vi "Push Digital.vi"(9 "Sample count":i32=8192, 10 "digital_samples":u64[](array[numeric]), 11 "ADALM2000 Handler":u32 caption="Instrument Handle Out") -> (3 "ADALM2000 Handler 2":u32 caption="Instrument Handle Out")   [LabVIEW 2015]
uses:
  libm2k_lv.dll
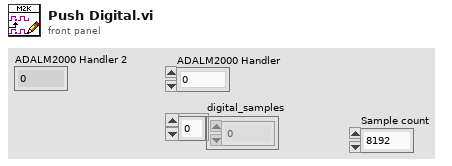
[diagram p1: front panel]
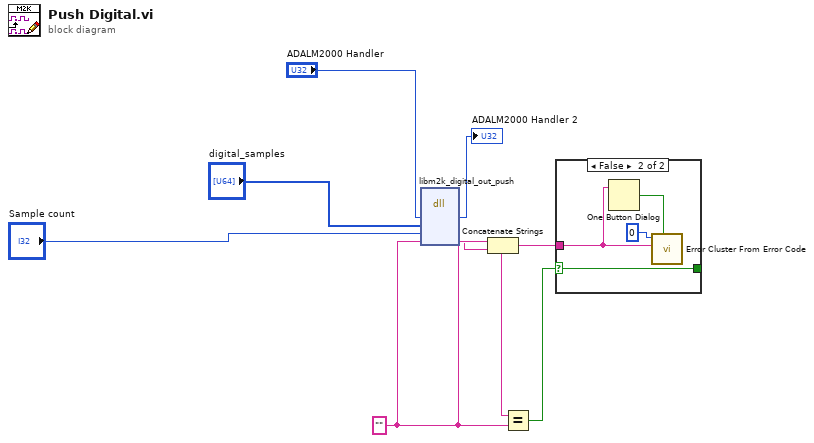
[diagram p0: block diagram]
diagram:
  w8 = ""
  n1 = dll-call lib="libm2k_lv.*" fn="libm2k_digital_out_push"("instance"="ADALM2000 Handler", "digital_samples"="digital_samples", "nb_samples"="Sample count", "err"=w8) -> ("instance"=→"ADALM2000 Handler 2":u64, "err"=w6:string)  [unwired: 6 in, 2 out]
  n2 = Concatenate Strings(w8, w6) -> (w4:string)
  n3 = Equal?(x=w4, y=w8) -> (x = y?=w5:bool)
  n4 = case shown="False" w5 {
    selector: w5 -> [w9 w10]
    tunnel: w4 -> [_ w12]
    tunnel: [w9 w10] -> _
    frame True {
    }
    frame False {
      n5 = One Button Dialog(message=w12) -> (true=w11:bool)  [unwired: 1 in]
      n6 = call <vilib>:"Error Cluster From Error Code.vi"("show call chain? (False)"=w11, "error message (\"\")"=w12, "error code (0)"=0) -> ()  [unwired: 6 in, 1 out]
    }
  }
